vi "Servo_serial_mac_readwrite2_2servo.vi"() -> ()   [LabVIEW 2017]
uses:
  <vilib>/Instr/_visa.llb/VISA Configure Serial Port (Instr).vi
panel:
  out "e Feedback":cluster{i32, dbl, dbl[]}(graph)
  out "Servo 2 Torque Feedback":cluster{i32, dbl, dbl[]}(graph)
  out "Servo 2 Position Feedback":cluster{i32, dbl, dbl[]}(graph)
  out "Servo 1 Torque Feedback":cluster{i32, dbl, dbl[]}(graph)
  out "Servo 1 Position Feedback":cluster{i32, dbl, dbl[]}(graph)
  out "Pos1 number":dbl
  out "Pos2 number":dbl
  out "Pos3 number":dbl
  out "Pos4 number":dbl
  out "Pos5 number":dbl
  in  "Delay":dbl
  in  "Buad Rate":i32(ring) items=["2400"=2400, "4800"=4800, "9600"=9600, "14400"=14400, "19200"=19200, "28800"=28800, "38400"=38400, "57600"=57600, "115200"=115200]
  out "Bytes at port":cluster{i32, dbl, dbl[]}(graph)
  out "Read from Arduino":string
  in  "Servo 5":dbl(knob) scale=0.0..180.0
  in  "Servo 4":dbl(knob) scale=0.0..180.0
  in  "Servo 3":dbl(knob) scale=0.0..180.0
  in  "Servo 2":dbl(knob) scale=0.0..180.0
  in  "Servo 1":dbl(knob) scale=0.0..180.0
  in  "stop":bool
  out "Sent to Arduino":string
  in  "COM Port":refnum<visa-resource-name>
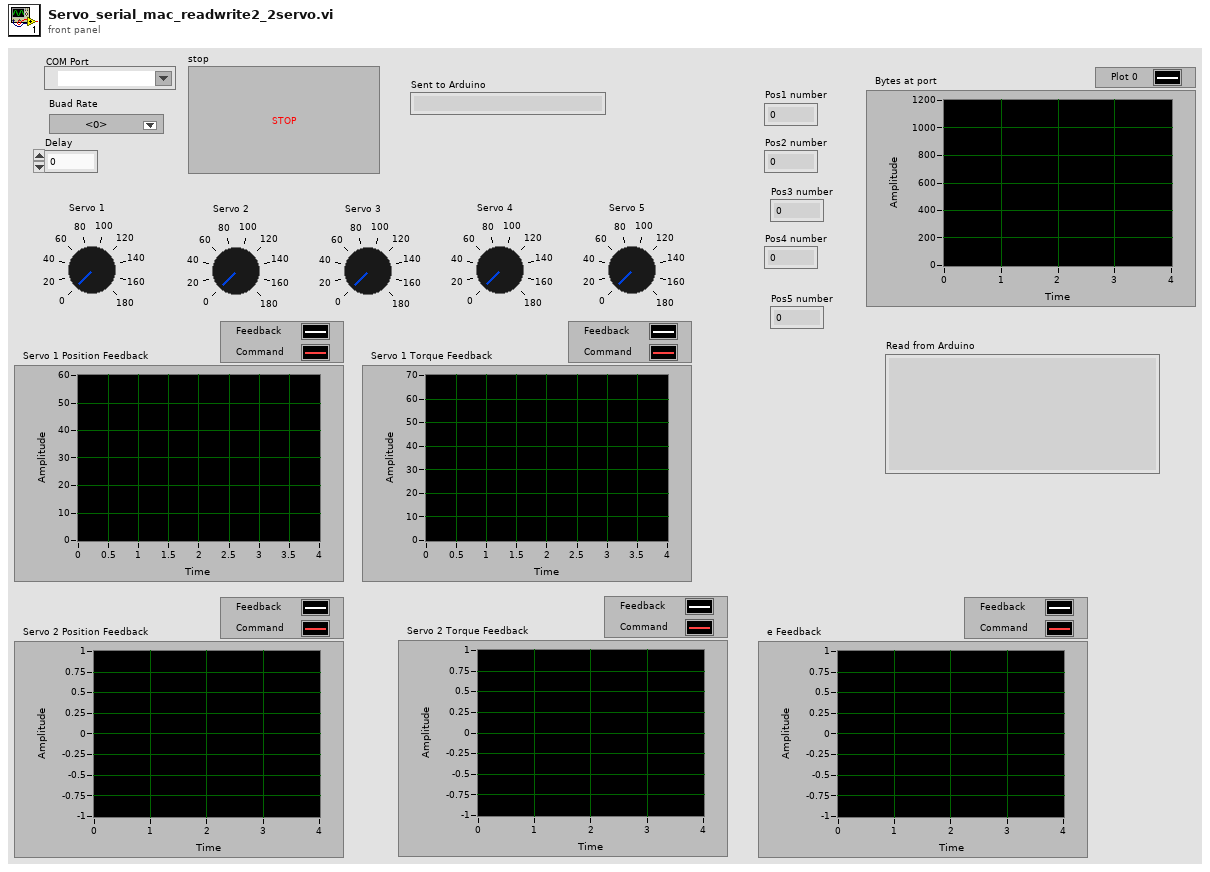
[diagram p1: front panel]
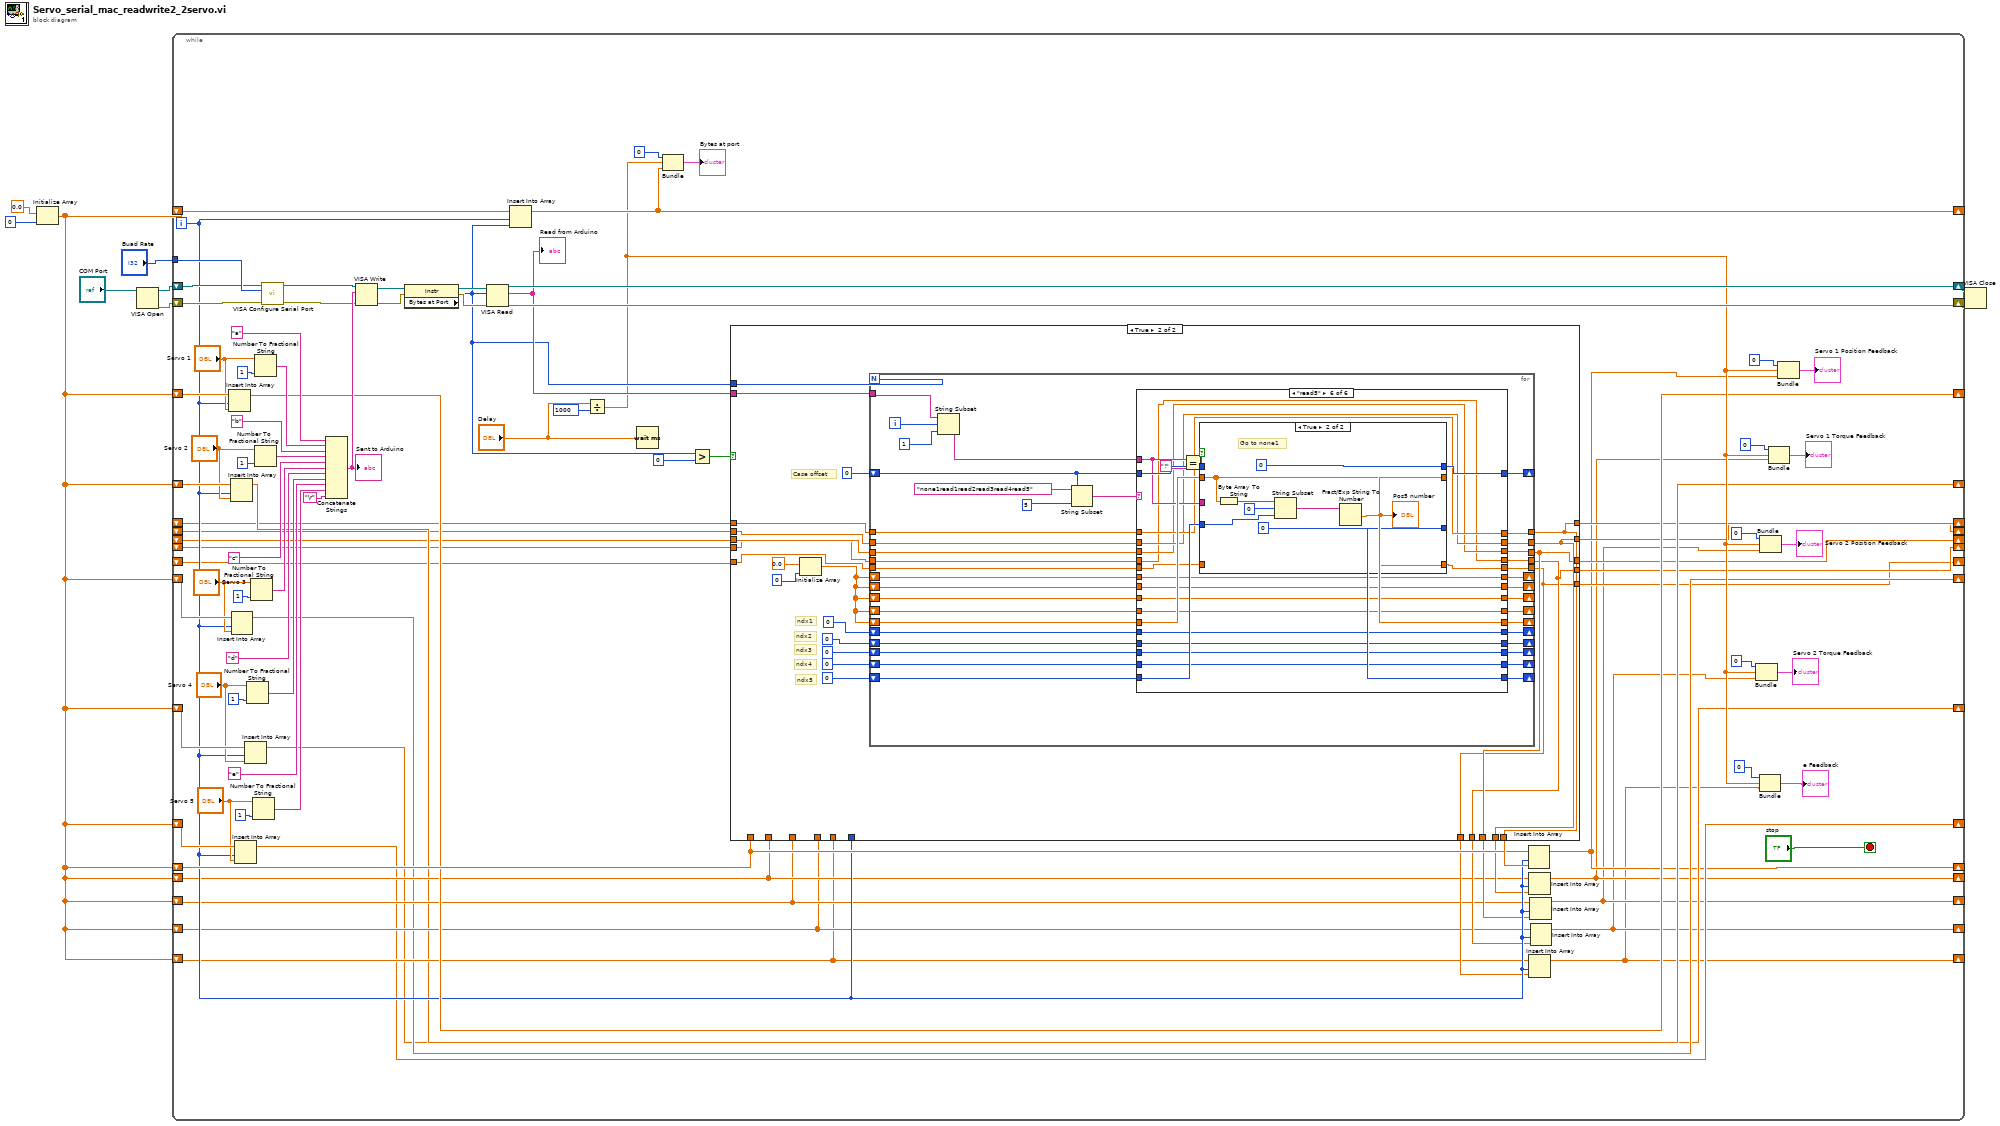
[diagram p0: block diagram]
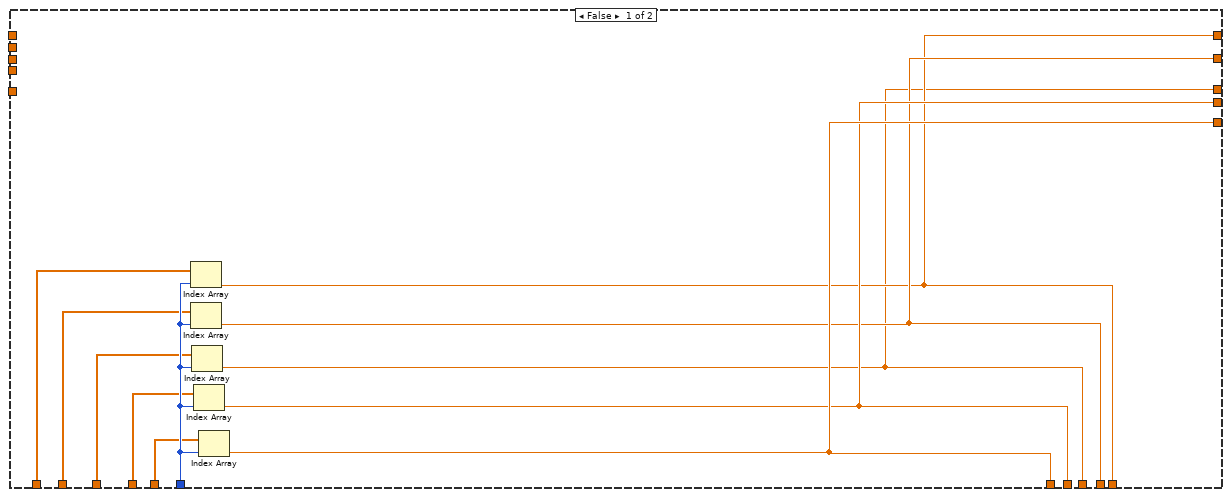
[diagram p2: hidden frame]
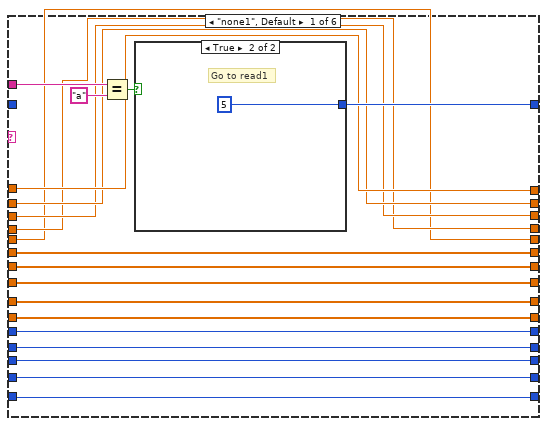
[diagram p3: hidden frame]
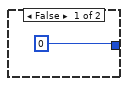
[diagram p4: hidden frame]
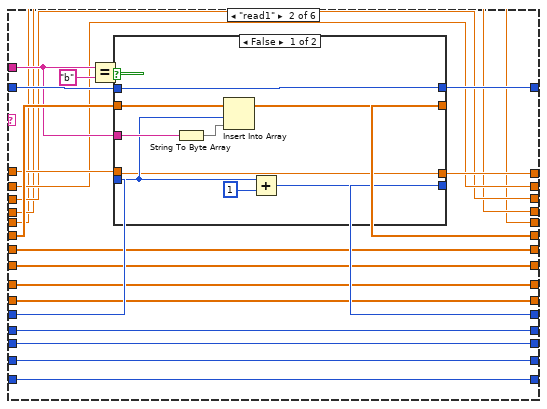
[diagram p5: hidden frame]
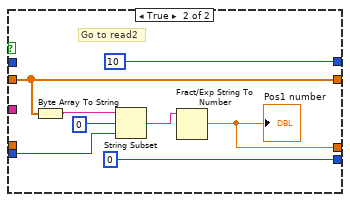
[diagram p6: hidden frame]
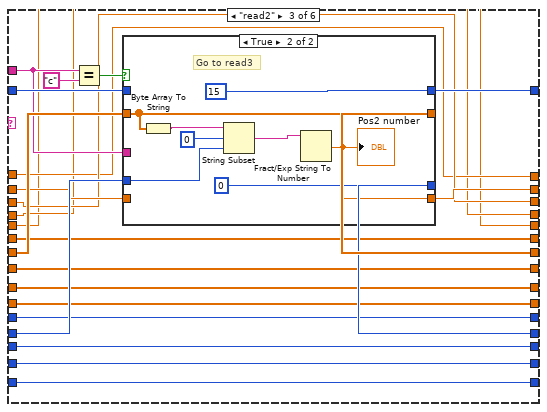
[diagram p7: hidden frame]
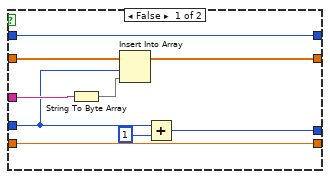
[diagram p8: hidden frame]
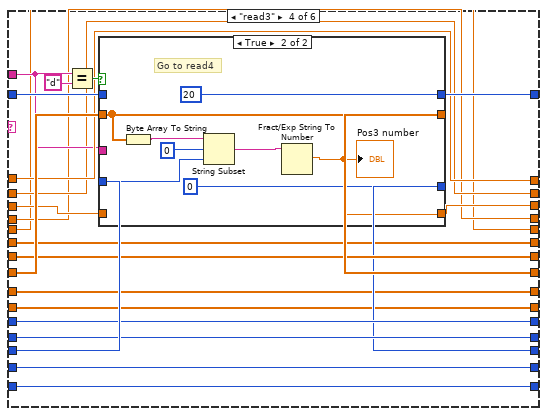
[diagram p9: hidden frame]
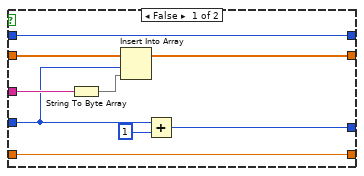
[diagram p10: hidden frame]
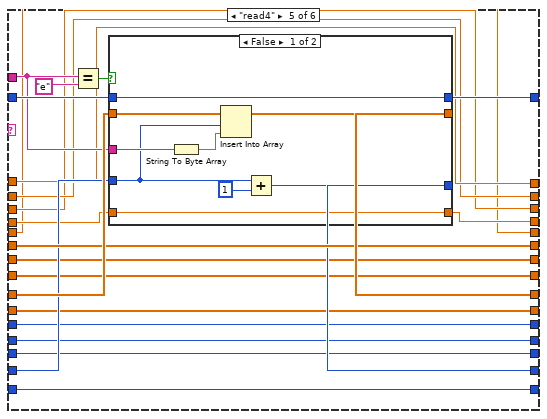
[diagram p11: hidden frame]
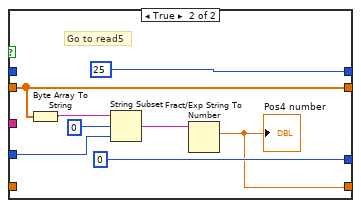
[diagram p12: hidden frame]
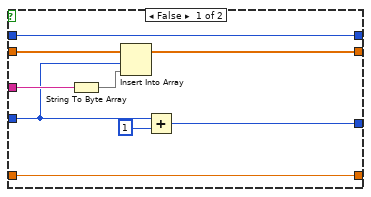
[diagram p13: hidden frame]
diagram:
  n1 = Initialize Array(0.0 ("element"), 0 ("dimension size")) -> (w1:dbl[])
  n2 = VISA Open(VISA resource name="COM Port") -> (VISA resource name=w8:refnum<visa-resource-name>, error out=w7:errorcluster)  [unwired: 4 in]
  n3 = while {
    tunnel: "Buad Rate" -> [w100]
    shift-right: [w96] -> w6
    shift-left: w8 -> [w99]
    shift-right: [w97] -> w5
    shift-left: w7 -> [w98]
    shift-right: [w94] -> _
    shift-left: w1 -> [w95]
    shift-right: [w38] -> _
    shift-left: w1 -> [w61]
    shift-right: [w28] -> _
    shift-left: w1 -> [w60]
    shift-right: [w27] -> _
    shift-left: w1 -> [w59]
    shift-right: [w26] -> _
    shift-left: w1 -> [w58]
    shift-right: [w25] -> _
    shift-left: w1 -> [w57]
    shift-right: [w14] -> _
    shift-left: w1 -> [w40]
    shift-right: [w13] -> _
    shift-left: w1 -> [w32]
    shift-right: [w12] -> _
    shift-left: w1 -> [w31]
    shift-right: [w11] -> _
    shift-left: w1 -> [w30]
    shift-right: [w10] -> _
    shift-left: w1 -> [w29]
    shift-right: [w19] -> _
    shift-left: _ -> [w24]
    shift-right: [w18] -> _
    shift-left: _ -> [w23]
    shift-right: [w17] -> _
    shift-left: _ -> [w22]
    shift-right: [w16] -> _
    shift-left: _ -> [w21]
    shift-right: [w15] -> _
    shift-left: _ -> [w20]
    i -> [w37]
    stop <- "stop" stop-if-true
    n4 = Insert Into Array(array=w61, index=w37, new element="Servo 1") -> (w38:dbl[])
    n5 = Insert Into Array(array=w60, index=w37, new element="Servo 2") -> (w28:dbl[])
    n6 = Insert Into Array(array=w59, index=w37, new element="Servo 3") -> (w27:dbl[])
    n7 = Insert Into Array(array=w57, index=w37, new element="Servo 5") -> (w25:dbl[])
    n8 = Insert Into Array(array=w58, index=w37, new element="Servo 4") -> (w26:dbl[])
    n9 = Number To Fractional String(number="Servo 4", precision (6)=1) -> (F-format string=w81:string)  [unwired: 2 in]
    n10 = Number To Fractional String(number="Servo 3", precision (6)=1) -> (F-format string=w88:string)  [unwired: 2 in]
    n11 = Number To Fractional String(number="Servo 5", precision (6)=1) -> (F-format string=w80:string)  [unwired: 2 in]
    n12 = Number To Fractional String(number="Servo 1", precision (6)=1) -> (F-format string=w90:string)  [unwired: 2 in]
    n13 = Number To Fractional String(number="Servo 2", precision (6)=1) -> (F-format string=w89:string)  [unwired: 2 in]
    n14 = call-poly "VISA Configure Serial Port"("VISA resource name"=w99, "baud rate (9600)"=w100, "error in (no error)"=w98) -> ("VISA resource name out"=w79:refnum<visa-resource-name>, "error out"=w91:errorcluster)  [unwired: 11 in]
    n15 = Concatenate Strings("a", w90, "b", w89, "c", w88, "d", w81, "e", w80, "\r") -> (w92:string)
    "Sent to Arduino" <- w92
    n16 = VISA Write(VISA resource name=w79, write buffer=w92, error in (no error)=w91) -> (VISA resource name out=w75:refnum<visa-resource-name>, error out=w78:errorcluster)  [unwired: 1 out]
    n17 = property class="Instr"(reference=w75, error in=w78) -> (reference out=w76:refnum<visa-resource-name>, error out=w77:errorcluster, "Bytes at Port"=w69:u32)
    n18 = VISA Read(VISA resource name=w76, byte count=w69, error in (no error)=w77) -> (VISA resource name out=w96:refnum<visa-resource-name>, read buffer=w71:string, error out=w97:errorcluster)  [unwired: 1 out]
    "Read from Arduino" <- w71
    n19 = Insert Into Array(array=w95, index=w37, new element=w69) -> (w94:dbl[])
    n20 = Divide(x="Delay", y=1000) -> (x/y=w39:dbl)
    n21 = Wait (ms)(milliseconds to wait="Delay") -> ()  [unwired: 1 out]
    n22 = Bundle(0, w39, w94) -> (→"Bytes at port":cluster{i32, dbl, dbl[]})  [unwired: 1 in]
    n23 = Greater?(x=w69, y=0) -> (0:w68:bool)
    n24 = case shown="True" w68 {
      tunnel: w69 -> [_ w122]
      tunnel: w71 -> [_ w132]
      tunnel: [w102 w116] -> w41
      tunnel: w37 -> [w110 _]
      tunnel: w40 -> [w111 _]
      tunnel: [w103 w115] -> w36
      tunnel: [w101 w114] -> w35
      tunnel: [w104 w113] -> w34
      tunnel: [w105 w112] -> w33
      tunnel: w32 -> [w109 _]
      tunnel: w31 -> [w108 _]
      tunnel: w30 -> [w107 _]
      tunnel: w29 -> [w106 _]
      tunnel: w24 -> [_ w121]
      tunnel: w23 -> [_ w120]
      tunnel: w22 -> [_ w119]
      tunnel: w21 -> [_ w118]
      tunnel: w20 -> [_ w117]
      tunnel: [w102 w116] -> w19
      tunnel: [w103 w115] -> w18
      tunnel: [w101 w114] -> w17
      tunnel: [w104 w113] -> w16
      tunnel: [w105 w112] -> w15
      frame False {
        n25 = Index Array(array=w111, index=w110) -> (element=w102:dbl)
        n26 = Index Array(array=w109, index=w110) -> (element=w103:dbl)
        n27 = Index Array(array=w108, index=w110) -> (element=w101:dbl)
        n28 = Index Array(array=w107, index=w110) -> (element=w104:dbl)
        n29 = Index Array(array=w106, index=w110) -> (element=w105:dbl)
      }
      frame True {
        # "ndx5"
        # "ndx4"
        # "ndx3"
        # "ndx2"
        # "ndx1"
        # "Case offset"
        n30 = Initialize Array(0.0 ("element"), 0 ("dimension size")) -> (w125:dbl[])
        n31 = for {
          N: w122 -> [_]
          tunnel: w132 -> [w170]
          shift-right: [w166] -> _
          shift-left: 0 -> [w157]
          shift-right: [w165] -> _
          shift-left: 0 -> [w164]
          shift-right: [w162] -> _
          shift-left: w125 -> [w163]
          shift-right: [w160] -> _
          shift-left: w125 -> [w161]
          shift-right: [w153] -> _
          shift-left: 0 -> [w159]
          shift-right: [w154] -> _
          shift-left: 0 -> [w155]
          shift-right: [w151] -> _
          shift-left: w125 -> [w152]
          shift-right: [w143] -> _
          shift-left: w125 -> [w150]
          shift-right: [w144] -> _
          shift-left: w125 -> [w149]
          shift-right: [w147] -> _
          shift-left: 0 -> [w148]
          shift-right: [w145] -> _
          shift-left: 0 -> [w146]
          tunnel: w121 -> [w141]
          tunnel: [w142] -> w116
          tunnel: w120 -> [w139]
          tunnel: [w140] -> w115
          tunnel: w119 -> [w137]
          tunnel: [w138] -> w114
          tunnel: w118 -> [w135]
          tunnel: [w136] -> w113
          tunnel: w117 -> [w133]
          tunnel: [w134] -> w112
          i -> [w156]
          n32 = String Subset(string=w170, offset (0)=w156, length (rest)=1 ("length (rest)")) -> (substring=w167:string)
          n33 = String Subset(string="none1read1read2read3read4read5", offset (0)=w157, length (rest)=5 ("length (rest)")) -> (substring=w158:string)
          n34 = case shown="\"read5\"" w158 {
            tunnel: w167 -> [w190 w209 w245 w279 w328 w369]
            tunnel: [w187 w212 w247 w287 w335 w372] -> w166
            tunnel: [w186 w207 w249 w292 w325 w362] -> w165
            tunnel: w164 -> [w186 w208 w249 w292 w325 w362]
            tunnel: w163 -> [w183 w210 w244 w273 w332 w366]
            tunnel: [w183 w213 w244 w273 w332 w366] -> w162
            tunnel: w161 -> [w184 w206 w255 w288 w323 w365]
            tunnel: [w184 w206 w254 w288 w323 w365] -> w160
            tunnel: w159 -> [w185 w202 w253 w291 w324 w361]
            tunnel: [w185 w202 w252 w291 w324 w361] -> w153
            tunnel: w157 -> [_ w211 w248 w294 w329 w371]
            tunnel: w155 -> [w180 w201 w246 w293 w320 w360]
            tunnel: [w180 w201 w246 w284 w320 w360] -> w154
            tunnel: w152 -> [w177 w205 w243 w290 w322 w364]
            tunnel: [w177 w205 w243 w289 w322 w364] -> w151
            tunnel: w150 -> [w178 w204 w242 w283 w334 w363]
            tunnel: w149 -> [w179 w203 w241 w282 w321 w374]
            tunnel: w148 -> [w182 w200 w240 w286 w327 w359]
            tunnel: [w182 w200 w240 w286 w326 w359] -> w147
            tunnel: w146 -> [w181 w199 w239 w285 w319 w368]
            tunnel: [w181 w199 w239 w285 w319 w367] -> w145
            tunnel: [w179 w203 w241 w282 w321 w373] -> w144
            tunnel: [w178 w204 w242 w283 w333 w363] -> w143
            tunnel: [w176 w198 w235 w281 w318 w358] -> w142
            tunnel: w141 -> [w176 w197 w235 w281 w318 w358]
            tunnel: [w175 w196 w238 w278 w317 w357] -> w140
            tunnel: w139 -> [w175 w196 w237 w278 w317 w357]
            tunnel: [w174 w195 w236 w277 w314 w355] -> w138
            tunnel: w137 -> [w174 w195 w236 w276 w314 w355]
            tunnel: [w173 w194 w234 w275 w316 w353] -> w136
            tunnel: w135 -> [w173 w194 w234 w275 w315 w353]
            tunnel: [w172 w193 w233 w274 w313 w356] -> w134
            tunnel: w133 -> [w172 w193 w233 w274 w313 w354]
            frame "none1", Default {
              n35 = Equal?(x=w190, y="a") -> (x = y?=w188:bool)
              n36 = case shown="True" w188 {
                tunnel: [0 5] -> w187
                frame False {
                }
                frame True {
                  # "Go to read1"
                }
              }
            }
            frame "read1" {
              n37 = Equal?(x=w209, y="b") -> (x = y?=w214:bool)
              n38 = case shown="False" w214 {
                tunnel: [w224 0] -> w207
                tunnel: w210 -> [w218 w228]
                tunnel: [w222 w228] -> w213
                tunnel: w209 -> [w221 _]
                tunnel: [w219 10] -> w212
                tunnel: w211 -> [w219 _]
                tunnel: w208 -> [w217 w227]
                tunnel: [w216 w225] -> w198
                tunnel: w197 -> [w216 _]
                frame False {
                  n39 = String To Byte Array(string=w221) -> (unsigned byte array=w220:u8[])
                  n40 = Insert Into Array(array=w218, index=w217, new element=w220) -> (w222:dbl[])
                  n41 = Add(x=w217, y=1) -> (x+y=w224:i32)
                }
                frame True {
                  # "Go to read2"
                  n42 = Byte Array To String(unsigned byte array=w228) -> (string=w229:string)
                  n43 = String Subset(string=w229, offset (0)=0, length (rest)=w227) -> (substring=w226:string)
                  n44 = Fract/Exp String To Number(string=w226) -> (number=w225:dbl)  [unwired: 3 in, 1 out]
                  "Pos1 number" <- w225
                }
              }
            }
            frame "read2" {
              n45 = Equal?(x=w245, y="c") -> (x = y?=w250:bool)
              n46 = case shown="True" w250 {
                tunnel: [w264 0] -> w252
                tunnel: w253 -> [w258 w269]
                tunnel: w255 -> [w262 w268]
                tunnel: [w261 w268] -> w254
                tunnel: w245 -> [w260 _]
                tunnel: [w257 15] -> w247
                tunnel: w248 -> [w257 _]
                tunnel: [w256 w265] -> w238
                tunnel: w237 -> [w256 _]
                frame False {
                  n47 = String To Byte Array(string=w260) -> (unsigned byte array=w259:u8[])
                  n48 = Insert Into Array(array=w262, index=w258, new element=w259) -> (w261:dbl[])
                  n49 = Add(x=w258, y=1) -> (x+y=w264:i32)
                }
                frame True {
                  # "Go to read3"
                  n50 = Byte Array To String(unsigned byte array=w268) -> (string=w267:string)
                  n51 = String Subset(string=w267, offset (0)=0, length (rest)=w269) -> (substring=w266:string)
                  n52 = Fract/Exp String To Number(string=w266) -> (number=w265:dbl)  [unwired: 3 in, 1 out]
                  "Pos2 number" <- w265
                }
              }
            }
            frame "read3" {
              n53 = Equal?(x=w279, y="d") -> (x = y?=w295:bool)
              n54 = case shown="True" w295 {
                tunnel: [w304 0] -> w284
                tunnel: w293 -> [w298 w307]
                tunnel: w290 -> [w302 w308]
                tunnel: [w301 w308] -> w289
                tunnel: w279 -> [w300 _]
                tunnel: [w297 20] -> w287
                tunnel: w294 -> [w297 _]
                tunnel: [w296 w305] -> w277
                tunnel: w276 -> [w296 _]
                frame False {
                  n55 = String To Byte Array(string=w300) -> (unsigned byte array=w299:u8[])
                  n56 = Insert Into Array(array=w302, index=w298, new element=w299) -> (w301:dbl[])
                  n57 = Add(x=w298, y=1) -> (x+y=w304:i32)
                }
                frame True {
                  # "Go to read4"
                  n58 = Byte Array To String(unsigned byte array=w308) -> (string=w309:string)
                  n59 = String Subset(string=w309, offset (0)=0, length (rest)=w307) -> (substring=w306:string)
                  n60 = Fract/Exp String To Number(string=w306) -> (number=w305:dbl)  [unwired: 3 in, 1 out]
                  "Pos3 number" <- w305
                }
              }
            }
            frame "read4" {
              n61 = Equal?(x=w328, y="e") -> (x = y?=w330:bool)
              n62 = case shown="False" w330 {
                tunnel: [w344 0] -> w326
                tunnel: w327 -> [w338 w347]
                tunnel: w334 -> [w342 w348]
                tunnel: [w341 w348] -> w333
                tunnel: w328 -> [w340 _]
                tunnel: [w337 25] -> w335
                tunnel: w329 -> [w337 _]
                tunnel: [w336 w345] -> w316
                tunnel: w315 -> [w336 _]
                frame False {
                  n63 = String To Byte Array(string=w340) -> (unsigned byte array=w339:u8[])
                  n64 = Insert Into Array(array=w342, index=w338, new element=w339) -> (w341:dbl[])
                  n65 = Add(x=w338, y=1) -> (x+y=w344:i32)
                }
                frame True {
                  # "Go to read5"
                  n66 = Byte Array To String(unsigned byte array=w348) -> (string=w349:string)
                  n67 = String Subset(string=w349, offset (0)=0, length (rest)=w347) -> (substring=w346:string)
                  n68 = Fract/Exp String To Number(string=w346) -> (number=w345:dbl)  [unwired: 3 in, 1 out]
                  "Pos4 number" <- w345
                }
              }
            }
            frame "read5" {
              n69 = Equal?(x=w369, y="!") -> (x = y?=w370:bool)
              n70 = case shown="True" w370 {
                tunnel: [w384 0] -> w367
                tunnel: w368 -> [w378 w387]
                tunnel: w374 -> [w382 w388]
                tunnel: [w381 w388] -> w373
                tunnel: w369 -> [w380 _]
                tunnel: [w377 0] -> w372
                tunnel: w371 -> [w377 _]
                tunnel: [w376 w385] -> w356
                tunnel: w354 -> [w376 _]
                frame False {
                  n71 = String To Byte Array(string=w380) -> (unsigned byte array=w379:u8[])
                  n72 = Insert Into Array(array=w382, index=w378, new element=w379) -> (w381:dbl[])
                  n73 = Add(x=w378, y=1) -> (x+y=w384:i32)
                }
                frame True {
                  # "Go to none1"
                  n74 = Byte Array To String(unsigned byte array=w388) -> (string=w389:string)
                  n75 = String Subset(string=w389, offset (0)=0, length (rest)=w387) -> (substring=w386:string)
                  n76 = Fract/Exp String To Number(string=w386) -> (number=w385:dbl)  [unwired: 3 in, 1 out]
                  "Pos5 number" <- w385
                }
              }
            }
          }
        }
      }
    }
    n77 = Insert Into Array(array=w40, index=w37, new element=w41) -> (w14:dbl[])
    n78 = Insert Into Array(array=w32, index=w37, new element=w36) -> (w13:dbl[])
    n79 = Insert Into Array(array=w29, index=w37, new element=w33) -> (w10:dbl[])
    n80 = Insert Into Array(array=w31, index=w37, new element=w35) -> (w12:dbl[])
    n81 = Insert Into Array(array=w30, index=w37, new element=w34) -> (w11:dbl[])
    n82 = Bundle(0, w39, w11) -> (→"Servo 2 Torque Feedback":cluster{i32, dbl, dbl[]})  [unwired: 1 in]
    n83 = Bundle(0, w39, w10) -> (→"e Feedback":cluster{i32, dbl, dbl[]})  [unwired: 1 in]
    n84 = Bundle(0, w39, w12) -> (→"Servo 2 Position Feedback":cluster{i32, dbl, dbl[]})  [unwired: 1 in]
    n85 = Bundle(0, w39, w13) -> (→"Servo 1 Torque Feedback":cluster{i32, dbl, dbl[]})  [unwired: 1 in]
    n86 = Bundle(0, w39, w14) -> (→"Servo 1 Position Feedback":cluster{i32, dbl, dbl[]})  [unwired: 1 in]
  }
  n87 = VISA Close(VISA resource name=w6, error in (no error)=w5) -> ()  [unwired: 1 out]
